vi "GetDataEventData.vi"(8 "error in (no error)":errorcluster, 11 "Data Value Reference in":T1) -> (0 "error out":errorcluster, 3 "Data":T2)   [LabVIEW 2017, in "DataEvent.lvlib"]
uses:
  <vilib>/addons/InsightCM/Devices/Shared/Common/DataEvent/DataEvent.lvlib
  <vilib>/addons/InsightCM/Devices/Shared/Common/DataEvent/controls/Event.ctl
  <vilib>/addons/InsightCM/MessageBus/Base/controls/DataEvent.ctl
  <vilib>/addons/InsightCM/MessageBus/Base/controls/KeyValuePair.ctl
  <vilib>/addons/InsightCM/Devices/Shared/Common/DataEvent/controls/DataSet.ctl
  <vilib>/addons/InsightCM/MessageBus/Base/controls/DataSetMetadata.ctl
  <vilib>/addons/InsightCM/MessageBus/Base/controls/TrendPoint.ctl
  <vilib>/addons/InsightCM/MessageBus/Base/controls/TrendAlarmUpdate.ctl
  <vilib>/addons/InsightCM/MessageBus/Base/controls/TrendAlarmTransition.ctl
  <vilib>/addons/InsightCM/Devices/Shared/Common/DataEvent/controls/EventReference.ctl
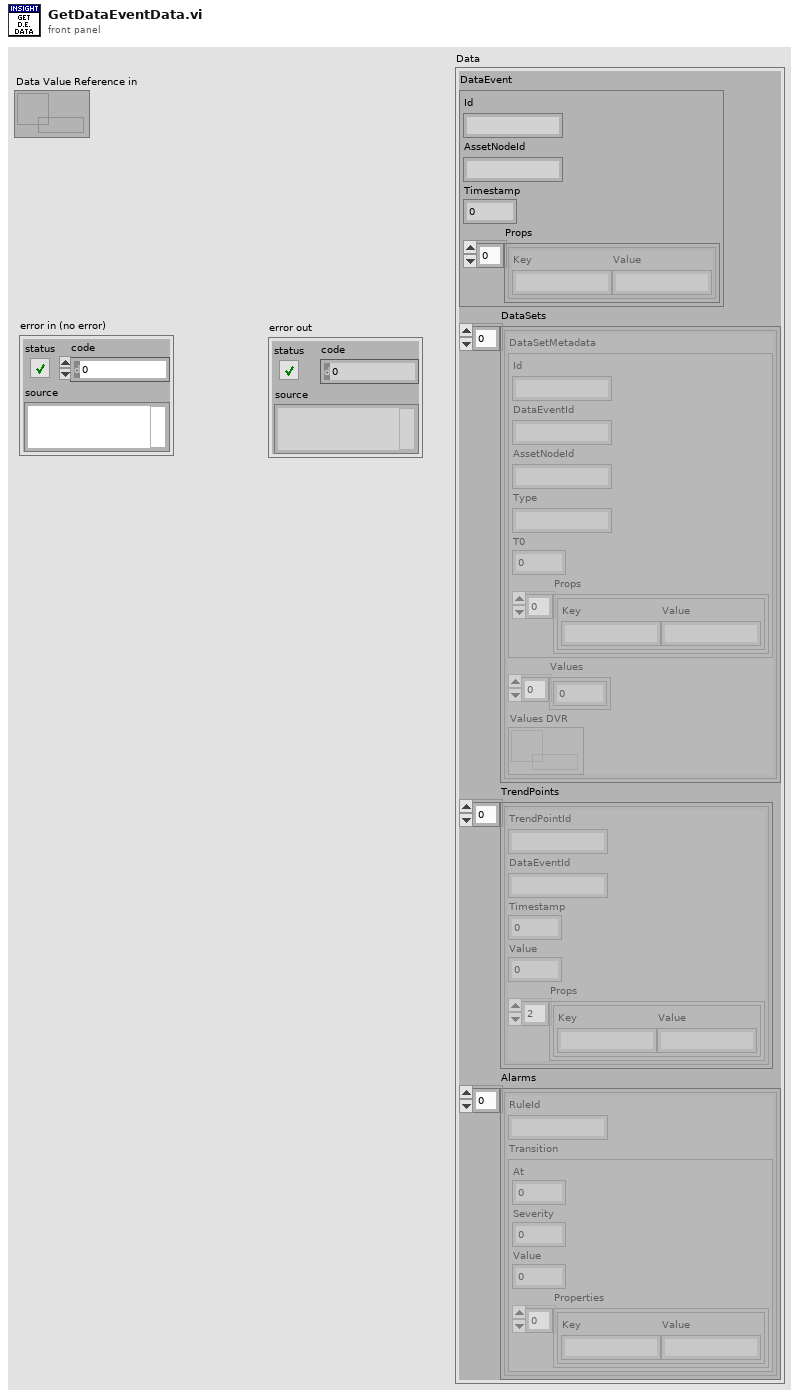
[diagram p1: front panel]
types:
  T1 = typedef "DataEvent.lvlib/EventReference.ctl" = refnum<data-value>
  T2 = typedef "DataEvent.lvlib/Event.ctl" = cluster{"DataEvent":T3, "DataSets":T5[], "TrendPoints":T7[], "Alarms":T8[]}
  T3 = typedef "DataEvent.ctl" = cluster{"Id":string, "AssetNodeId":string, "Timestamp":i64, "Props":T4[]}
  T4 = typedef "KeyValuePair.ctl" = cluster{"Key":string, "Value":string}
  T5 = typedef "DataEvent.lvlib/DataSet.ctl" = cluster{"DataSetMetadata":T6, "Values":sgl[], "Values DVR":refnum<data-value>}
  T6 = typedef "DataSetMetadata.ctl" = cluster{"Id":string, "DataEventId":string, "AssetNodeId":string, "Type":string, "T0":i64, "Props":T4[]}
  T7 = typedef "TrendPoint.ctl" = cluster{"TrendPointId":string, "DataEventId":string, "Timestamp":i64, "Value":dbl, "Props":T4[]}
  T8 = typedef "TrendAlarmUpdate.ctl" = cluster{"RuleId":string, "Transition":T9}
  T9 = typedef "TrendAlarmTransition.ctl" = cluster{"At":i64, "Severity":i32, "Value":dbl, "Properties":T4[]}
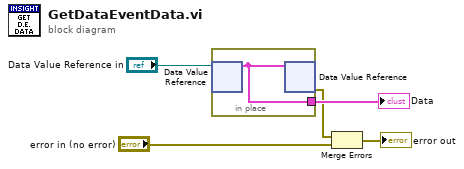
[diagram p0: block diagram]
diagram:
  n1 = in-place {
    in-place-border: [w6] -> w5
    n2 = in-place-dvr #1("Data Value Reference in") -> (w6:T2)  [unwired: 1 out]
    n3 = in-place-dvr #1(w6) -> (w3:errorcluster)  [unwired: 1 out]
  }
  "Data" <- w5
  n4 = Merge Errors(w3, "error in (no error)") -> (→"error out":errorcluster)
